vi "FROG_average_2.vi"() -> ()   [LabVIEW 2016]
uses:
  <vilib>/Utility/file.llb/Write Delimited Spreadsheet (DBL).vi
  <instrlib>/Ocean Optics 2000 4000/Ocean Optics 2000 4000.lvlib
panel:
  in  "Save FROG? 2":bool
  in  "Stop\nFROG NOW":bool=TRUE
  out "Spectral Waveform 2":cluster{dbl[], dbl[]}(graph)
  in  "Start FROG 2":bool
  in  "Integration Time (6000us)":u32=6000
  in  "Average #":i32=5
  out "0.5*Max intens":dbl=903.2
  in  "Final Position, mm":ext=13.501
  out "Pulse":dbl[][](graph)
  in  "Enable Strobe (Disabled)":bool
  in  "VISA resource name":refnum<visa-resource-name>="USB0::0x2457::0x1012::NI-VISA-10001::RAW"
  in  "Initial Position, mm":ext=13.5
  in  "Step Size, mm":ext=0.0001
  in  "MG17Motor":refnum<k7>(container)
  # "1st save is spectrogram itself,  2nd save is xy axes"
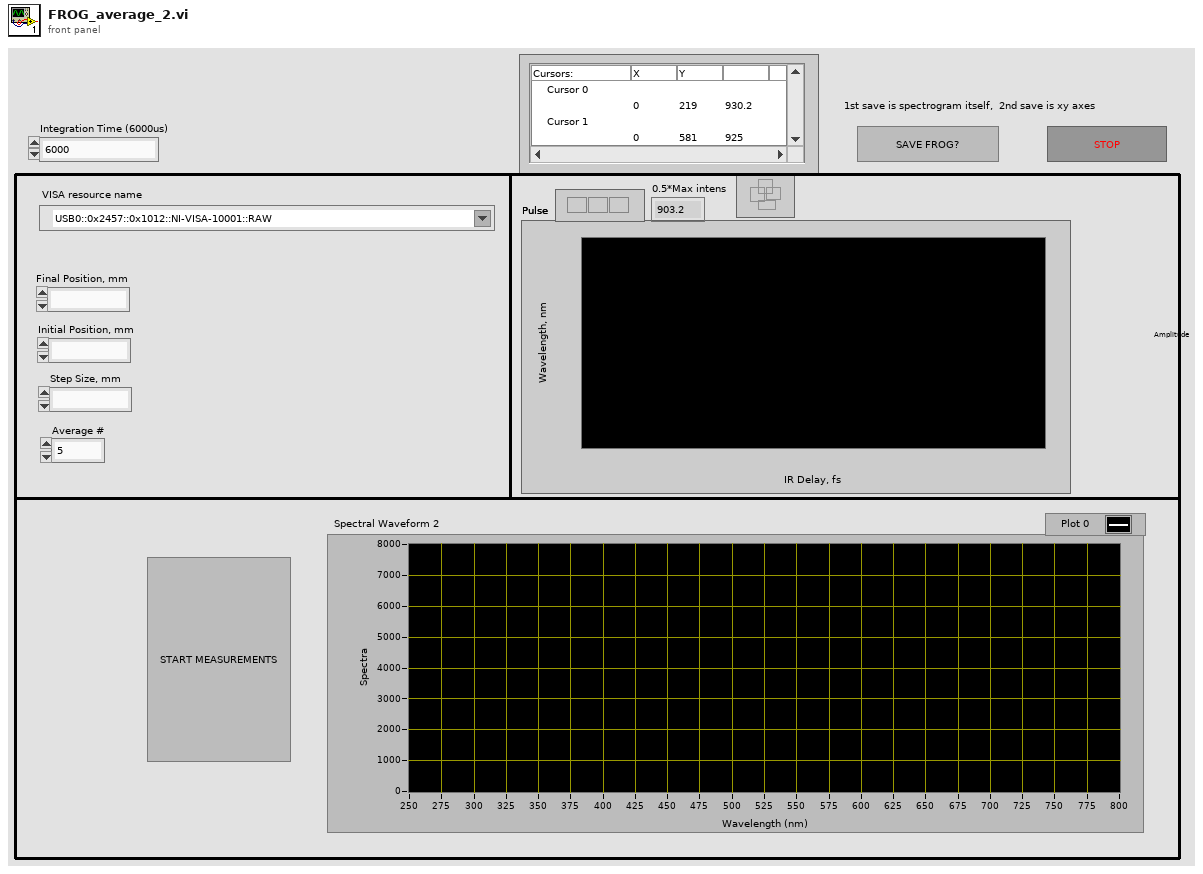
[diagram p1: front panel]
types:
  T1 = cluster{"Wavelength (nm)":dbl[], "Spectrum by Pixel Number":dbl[]}
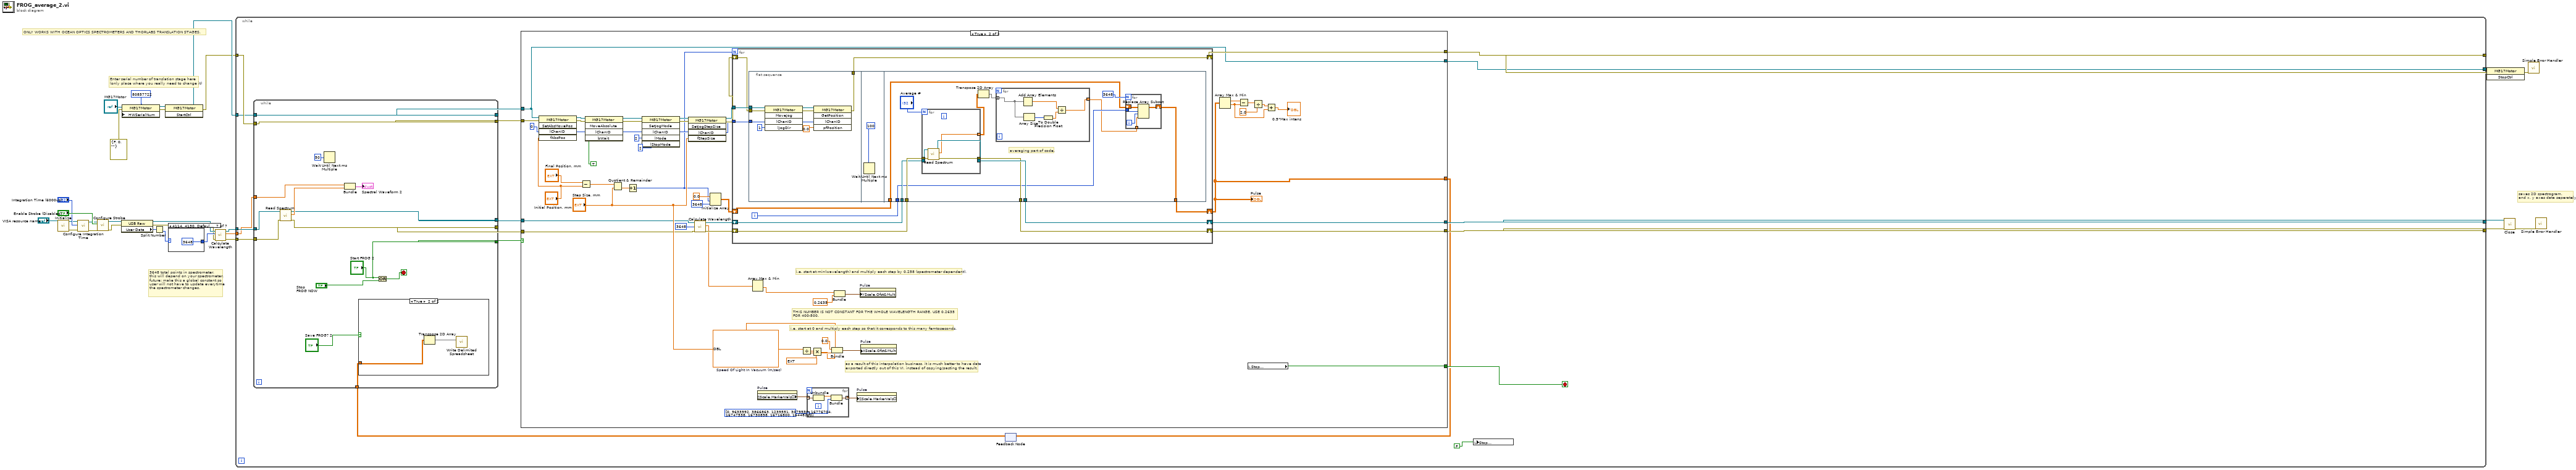
[diagram p0: block diagram]
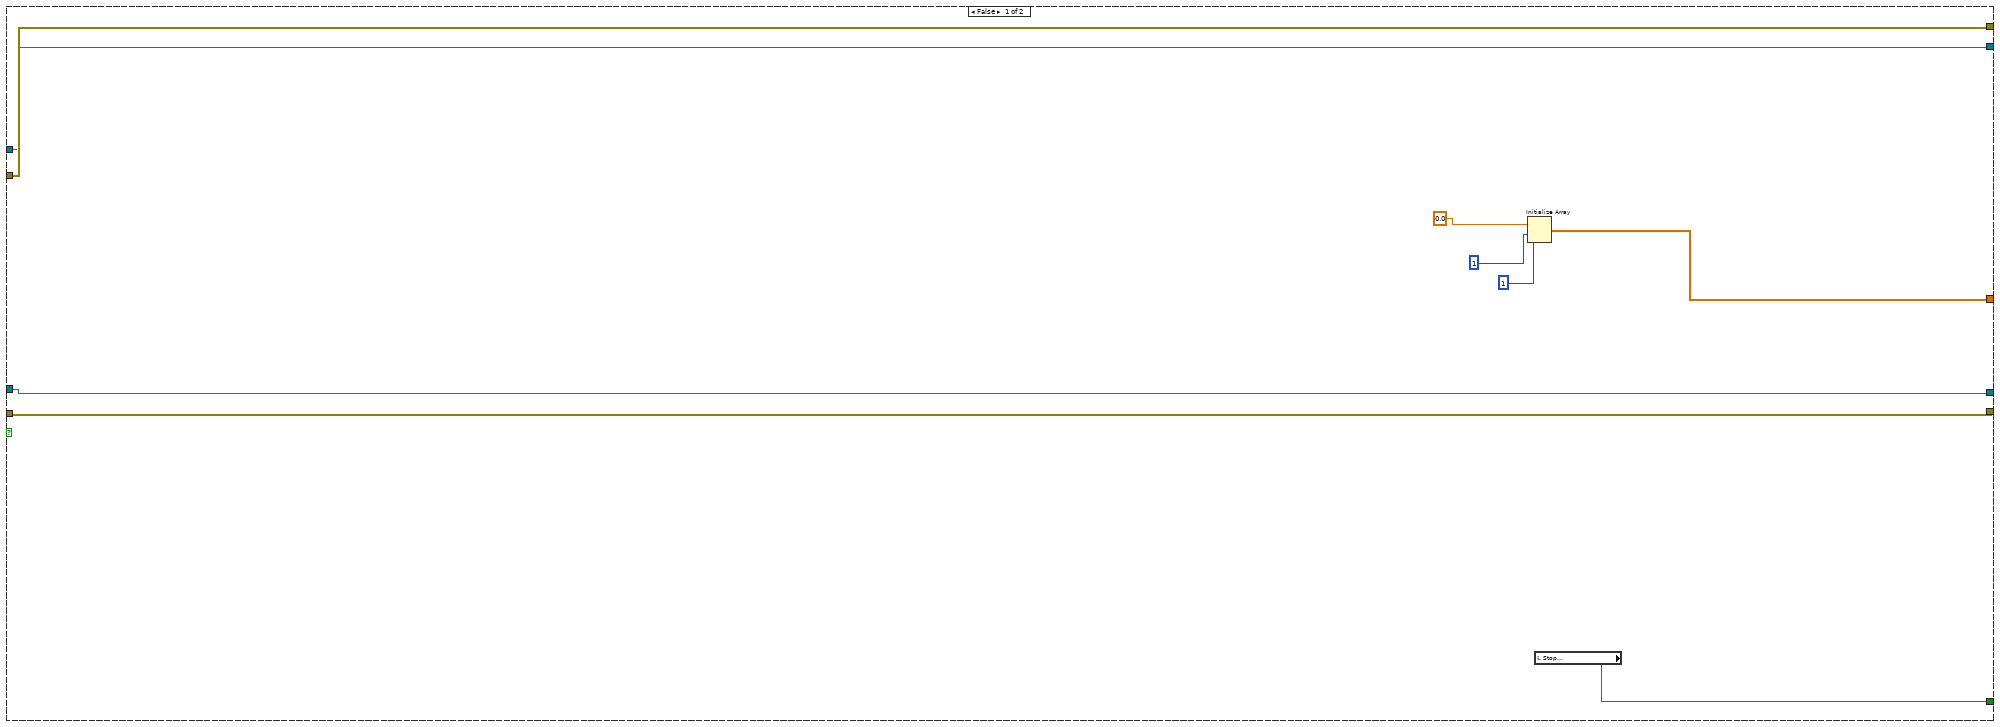
[diagram p2: hidden frame]
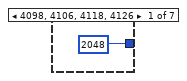
[diagram p4: hidden frame]
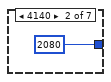
[diagram p5: hidden frame]
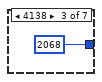
[diagram p6: hidden frame]
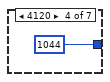
[diagram p7: hidden frame]
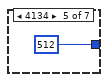
[diagram p8: hidden frame]
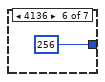
[diagram p9: hidden frame]
diagram:
  # "saves 2D spectrogram,\nand x, y axes data seperately."
  # "ONLY WORKS WITH OCEAN OPTICS SPECTROMETERS AND THORLABS TRANSLATION STAGES."
  # "3648 total points in spectrometer,\nthis will depend on your spectrometer.\nfuture: make this a global constant so \nuser will not have to update everytime\nthe spectrometer changes."
  # "Enter serial number of translation stage here\n(only place where you really need to change it)"
  n1 = call <instrlib>:"Initialize.vi"("VISA resource name"="VISA resource name") -> ("error out"=w9:errorcluster, "VISA resource name out"=w10:refnum<visa-resource-name>)  [unwired: 2 in, 7 out]
  n2 = call <instrlib>:"Configure Integration Time.vi"("error in (no error)"=w9, "Integration Time (6000)"="Integration Time (6000us)", "VISA resource name"=w10) -> ("error out"=w8:errorcluster, "VISA resource name out"=w7:refnum<visa-resource-name>)  [unwired: 7 out]
  n3 = call <instrlib>:"Configure Strobe.vi"("error in (no error)"=w8, "Enable Strobe (Disabled)"="Enable Strobe (Disabled)", "VISA resource name"=w7) -> ("error out"=w19:errorcluster, "VISA resource name out"=w18:refnum<visa-resource-name>)  [unwired: 7 out]
  n4 = property class="USB Raw"(reference=w18, error in=w19) -> (reference out=w16:refnum<visa-resource-name>, error out=w15:errorcluster, "User Data"=w24:u32)
  n5 = property class="MG17Motor"(reference="MG17Motor", error in=errorcluster {"status"=FALSE, "code"=0, "source"=""} ("error in (no error)"), "HWSerialNum"=80857722) -> (reference out=w28:refnum<k7>, error out=w27:errorcluster)
  n6 = Split Number(x=w24) -> (lo(x)=w23:u16)  [unwired: 1 out]
  n7 = invoke class="MG17Motor" method="StartCtrl"(reference=w28, error in=w27) -> (reference out=w6:refnum<k7>, error out=w5:errorcluster)  [unwired: 1 in, 1 out]
  n8 = case shown="4114, 4130, Default" w23 {
    tunnel: [2048 ("Number of Pixels (3840)") 2080 ("Number of Pixels (3840)") 2068 ("Number of Pixels (3840)") 1044 ("Number of Pixels (3840)") 512 ("Number of Pixels (3840)") 256 ("Number of Pixels (3840)") 3648 ("Number of Pixels (3840)")] -> w17
    frame 4098, 4106, 4118, 4126 {
    }
    frame 4140 {
    }
    frame 4138 {
    }
    frame 4120 {
    }
    frame 4134 {
    }
    frame 4136 {
    }
    frame 4114, 4130, Default {
    }
  }
  n9 = call <instrlib>:"Calculate Wavelength.vi"("error in (no error)"=w15, "Number of Pixels (3648)"=w17, "VISA resource name"=w16) -> ("error out"=w3:errorcluster, "Wavelength (nm)"=w2:dbl[], "VISA resource name out"=w4:refnum<visa-resource-name>)  [unwired: 6 out]
  n10 = while {
    tunnel: w6 -> [w48]
    tunnel: [w54] -> w14
    tunnel: [w53] -> w13
    tunnel: w4 -> [w52]
    tunnel: w3 -> [w51]
    tunnel: w2 -> [w50]
    tunnel: [w43] -> w1
    tunnel: w5 -> [w49]
    tunnel: [w55] -> w25
    stop <- w40 stop-if-true
    n11 = feedback #1() -> (w38:dbl[][])  [unwired: 1 in]
    n12 = while {
      tunnel: w52 -> [w181]
      tunnel: w50 -> [w182]
      tunnel: [w179] -> w45
      tunnel: [w178] -> w44
      tunnel: w51 -> [w180]
      tunnel: w49 -> [w186]
      tunnel: w48 -> [w187]
      tunnel: [w187] -> w47
      tunnel: [w186] -> w46
      tunnel: ["Start FROG 2"] -> w42
      tunnel: w38 -> [w173]
      stop <- w177 stop-if-true
      n13 = call <instrlib>:"Read Spectrum.vi"("error in (no error)"=w180, "VISA resource name"=w181) -> ("error out"=w178:errorcluster, "Spectrum by Pixel Number"=w183:dbl[], "VISA resource name out"=w179:refnum<visa-resource-name>)  [unwired: 6 in, 1 out]
      n14 = Wait Until Next ms Multiple(millisecond multiple=u32 50) -> ()  [unwired: 1 out]
      n15 = Bundle("Wavelength (nm)"=w182, "Spectrum by Pixel Number"=w183) -> (→"Spectral Waveform 2":T1)  [unwired: 1 out]
      n16 = case shown="True" "Save FROG? 2" {
        tunnel: w173 -> [_ w188]
        frame False {
        }
        frame True {
          n17 = Transpose 2D Array(2D array=w188) -> (transposed array=w189:dbl[][])
          n18 = call-poly <vilib>:"Write Delimited Spreadsheet.vi"("2D data"=w189) -> ()  [unwired: 13 in, 2 out]
        }
      }
      n19 = Or(x="Start FROG 2", y="Stop\nFROG NOW") -> (x .or. y?=w177:bool)
    }
    n20 = case shown="True" w42 {
      tunnel: [w64 w103] -> w55
      tunnel: [w62 w81] -> w54
      tunnel: [w61 w80] -> w53
      tunnel: w47 -> [w63 w70]
      tunnel: w46 -> [w64 w76]
      tunnel: w45 -> [w62 w75]
      tunnel: w44 -> [w61 w74]
      tunnel: [w63 w70] -> w43
      tunnel: [w59 w65] -> w39
      tunnel: [w58 w66] -> w40
      frame False {
        n21 = Initialize Array(0.0, 1, 1) -> (w59:dbl[][])
        n22 = local read "Stop\nFROG NOW"() -> (w58:bool)
      }
      frame True {
        w119 = ext[unit] 299792458.0  # Speed Of Light In Vacuum (m/sec)
        # "as a result of this interpolation business, it is much better to have data\nexported directly out of this VI, instead of copying/pasting the result."
        # "THIS NUMBER IS NOT CONSTANT FOR THE WHOLE WAVELENGTH RANGE. USE 0.2635\nFOR 400-500."
        # "i.e. start at min(wavelength) and multiply each step by 0.258 (spectrometer dependent)."
        # "i.e. start at 0 and multiply each step so that it corresponds to this many femtoseconds."
        n23 = invoke class="MG17Motor" method="SetAbsMovePos"(reference=w70, error in=w76, "lChanID"=0, "fAbsPos"="Initial Position, mm") -> (reference out=w105:refnum<k7>, error out=w104:errorcluster, "lChanID"=w102:i32)  [unwired: 1 in, 2 out]
        n24 = Subtract(x="Final Position, mm", y="Initial Position, mm") -> (x-y=w92:ext)
        n25 = invoke class="MG17Motor" method="MoveAbsolute"(reference=w105, error in=w104, "lChanID"=w102, "bWait"=TRUE) -> (reference out=w96:refnum<k7>, error out=w95:errorcluster, "lChanID"=w101:i32)  [unwired: 1 in, 2 out]
        n26 = Quotient & Remainder(x=w92, y="Step Size, mm") -> (floor(x/y)=w91:ext)  [unwired: 1 out]
        n27 = Increment(x=w91) -> (x+1=w67:i32)
        n28 = invoke class="MG17Motor" method="SetJogMode"(reference=w96, error in=w95, "lChanID"=w101, "lMode"=2, "lStopMode"=2) -> (reference out=w110:refnum<k7>, error out=w108:errorcluster, "lChanID"=w100:i32)  [unwired: 1 in, 3 out]
        n29 = invoke class="MG17Motor" method="SetJogStepSize"(reference=w110, error in=w108, "lChanID"=w100, "fStepSize"="Step Size, mm") -> (reference out=w109:refnum<k7>, error out=w107:errorcluster, "lChanID"=w99:i32)  [unwired: 1 in, 2 out]
        n30 = call <instrlib>:"Calculate Wavelength.vi"("error in (no error)"=w74, "Number of Pixels (3648)"=3648, "VISA resource name"=w75) -> ("error out"=w82:errorcluster, "Wavelength (nm)"=w68:dbl[], "VISA resource name out"=w83:refnum<visa-resource-name>)  [unwired: 6 out]
        n31 = Initialize Array(0.0 ("element"), w67, 3648 ("dimension size")) -> (w88:dbl[][])
        n32 = for {
          N: w67 -> [_]
          tunnel: w109 -> [w135]
          tunnel: w99 -> [w133]
          shift-right: [w129] -> w81
          shift-left: w83 -> [w132]
          shift-right: [w128] -> w80
          shift-left: w82 -> [w131]
          shift-right: [w125] -> w65
          shift-left: w88 -> [w127]
          shift-right: [w130] -> w103
          shift-left: w107 -> [w134]
          i -> [w126]
          n33 = flat-sequence {
            tunnel: w135 -> [w139]
            tunnel: w134 -> [w138]
            tunnel: w133 -> [w137]
            tunnel: [w136] -> w130
            tunnel: w132 -> [w153]
            tunnel: w131 -> [w154]
            tunnel: [w151] -> w128
            tunnel: [w152] -> w129
            tunnel: w126 -> [w150]
            tunnel: w127 -> [w156]
            tunnel: [w155] -> w125
            frame #0 {
              n34 = invoke class="MG17Motor" method="MoveJog"(reference=w139, error in=w138, "lChanID"=w137, "lJogDir"=1) -> (reference out=w143:refnum<k7>, error out=w144:errorcluster, "lChanID"=w140:i32)  [unwired: 1 in, 2 out]
              n35 = invoke class="MG17Motor" method="GetPosition"(reference=w143, error in=w144, "lChanID"=w140, "pfPosition"=sgl 0.0) -> (error out=w136:errorcluster)  [unwired: 1 in, 4 out]
            }
            frame #1 {
              n36 = Wait Until Next ms Multiple(millisecond multiple=u32 100) -> ()  [unwired: 1 out]
            }
            frame #2 {
              # "averaging part of code."
              n37 = for {
                N: "Average #" -> [_]
                tunnel: [w163] -> w148 mode=indexing
                tunnel: w154 -> [w167]
                tunnel: [w164] -> w151
                tunnel: w153 -> [w166]
                tunnel: [w165] -> w152
                n38 = call <instrlib>:"Read Spectrum.vi"("error in (no error)"=w167, "VISA resource name"=w166) -> ("error out"=w164:errorcluster, "Spectrum by Pixel Number"=w163:dbl[], "VISA resource name out"=w165:refnum<visa-resource-name>)  [unwired: 6 in, 1 out]
              }
              n39 = Transpose 2D Array(2D array=w148) -> (transposed array=w147:dbl[][])
              n40 = for {
                tunnel: [w159] -> w146 mode=indexing
                tunnel: w147 -> [w158] mode=indexing
                n41 = Add Array Elements(numeric array=w158) -> (sum=w160:dbl)
                n42 = Array Size(array=w158) -> (size(s)=w162:i32)
                n43 = To Double Precision Float(number=w162) -> (double precision float=w161:dbl)
                n44 = Divide(x=w160, y=w161) -> (x/y=w159:dbl)
              }
              n45 = for {
                N: 3648 -> [_]
                shift-right: [w171] -> w155
                shift-left: w156 -> [w172]
                tunnel: w150 -> [w168]
                tunnel: w146 -> [w170] mode=indexing
                i -> [w169]
                n46 = Replace Array Subset(array=w172, new element=w170, index (row)=w168, index (col)=w169) -> (w171:dbl[][])
              }
            }
          }
        }
        "Pulse" <- w65
        n47 = Array Max & Min(array=w68) -> (min value=w79:dbl)  [unwired: 3 out]
        n48 = property on="Pulse" class="IntGraph (strict)"() -> ("ZScale.MarkerVals[]"=w113:cluster{dbl, u32}[])  [unwired: 2 in, 2 out]
        n49 = Divide(x="Step Size, mm", y=w119) -> (x/y=w118:ext)
        n50 = for {
          tunnel: w113 -> [w124] mode=indexing
          tunnel: u32[] [0, 9633992, 3866863, 1239551, 3079936, 16776704, 16747538, 16730898, 16716800, 16448250] ("Custom Marker Colors 2") -> [w122] mode=indexing
          tunnel: [w121] -> w112 mode=indexing
          n51 = Unbundle(w124) -> (w123:dbl)  [unwired: 1 out]
          n52 = Bundle(w123, "Color Box"=w122) -> (w121:cluster{dbl, "Color Box":u32})  [unwired: 1 in]
        }
        n53 = Multiply(x=w118, y=ext 2000000000000.0) -> (x*y=w69:ext)
        n54 = Bundle(0.0, w69) -> (w115:cluster{dbl, ext})  [unwired: 1 in]
        n55 = Bundle(w79, 0.2635) -> (w120:cluster{dbl, dbl})  [unwired: 1 in]
        n56 = property on="Pulse" class="IntGraph (strict)"("ZScale.MarkerVals[]"=w112) -> ()  [unwired: 2 in, 2 out]
        n57 = property on="Pulse" class="IntGraph (strict)"("YScale.Ofst&Mult"=w120) -> ()  [unwired: 2 in, 2 out]
        n58 = property on="Pulse" class="IntGraph (strict)"("XScale.Ofst&Mult"=w115) -> ()  [unwired: 2 in, 2 out]
        n59 = Array Max & Min(array=w65) -> (max value=w87:dbl, min value=w71:dbl)  [unwired: 2 out]
        n60 = Subtract(x=w87, y=w71) -> (x-y=w86:dbl)
        n61 = local read "Stop\nFROG NOW"() -> (w66:bool)
        n62 = Divide(x=w86, y=2.0) -> (x/y=w72:dbl)
        n63 = Add(x=w72, y=w71) -> (x+y=→"0.5*Max intens":dbl)
      }
    }
    n64 = feedback-in #1(w39) -> ()
    n65 = local write "Stop\nFROG NOW"(FALSE) -> ()
  }
  n66 = invoke class="MG17Motor" method="StopCtrl"(reference=w1, error in=w25) -> (error out=w22:errorcluster)  [unwired: 1 in, 2 out]
  n67 = call <instrlib>:"Close.vi"("error in (no error)"=w13, "VISA resource name"=w14) -> ("error out"=w12:errorcluster)  [unwired: 9 out]
  n68 = call <vilib>:"Simple Error Handler.vi"("error in (no error)"=w22) -> ()  [unwired: 1 in, 8 out]
  n69 = call <vilib>:"Simple Error Handler.vi"("error in (no error)"=w12) -> ()  [unwired: 1 in, 8 out]
